vi "RT Loop - Watchdog.vi"(10 "FPGA VI Reference":T1, 11 "Message Queue":refnum<queue>) -> ()   [LabVIEW 2018]
uses:
  support/Message Queue/Message Cluster.ctl
  controls/FPGA VI Reference.ctl
  Globals/Global - Configuration Options.vi
  <vilib>/Utility/error.llb/Error Cluster From Error Code.vi
  <vilib>/rvi/errors/niLvFpgaAdjustHostInterfaceError.vi
  Globals/Global - All RT Loop Stop.vi
  <vilib>/rvi/interface/nirviReadWriteControl/nirviReadWriteControl.xnode
  NiFpgaLv.dll
  <vilib>/rvi/interface/Simulation/niFpgaSimulationCallBeginRW.vi
  support/Message Queue/Message Queue.lvlib
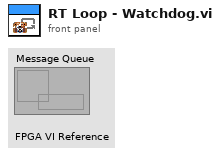
[diagram p1: front panel]
types:
  T1 = typedef "FPGA VI Reference.ctl" = refnum<k20>
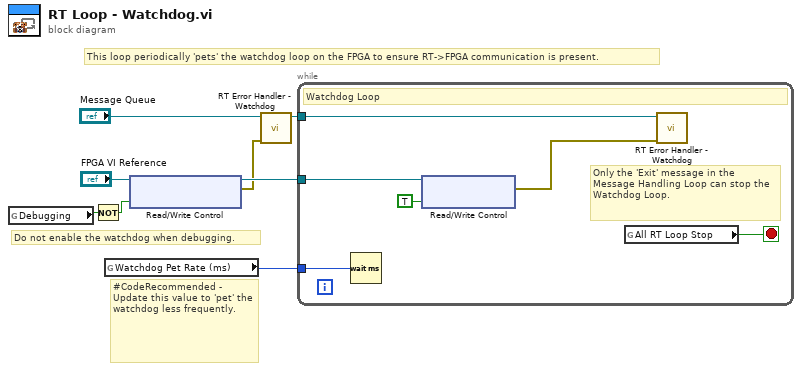
[diagram p0: block diagram]
diagram:
  # "Do not enable the watchdog when debugging."
  # "#CodeRecommended - Update this value to 'pet' the watchdog less frequently."
  # "This loop periodically 'pets' the watchdog loop on the FPGA to ensure RT->FPGA communication is present."
  n1 = global read "Global - Configuration Options.vi" "Debugging"() -> (w2:bool)
  n2 = Not(x=w2) -> (.not. x?=w1:bool)
  n3 = global read "Global - Configuration Options.vi" "Watchdog Pet Rate (ms)"() -> (w8:u32)
  n4 = xnode "Read/Write Control"("FPGA VI Reference In"="FPGA VI Reference", "Enable Watchdog"=w1) -> ("FPGA VI Reference Out"=w6:T1, "error out"=w3:errorcluster)  [unwired: 1 in]
  n5 = call "RT Error Handler - Watchdog.vi"("error in (no error)"=w3, "Message Queue"="Message Queue") -> ("dup Message Queue"=w4:refnum<queue>)  [unwired: 9 in]
  n6 = while {
    tunnel: w4 -> [w11]
    tunnel: w6 -> [w14]
    tunnel: w8 -> [w9]
    stop <- w12 stop-if-true
    # "Only the 'Exit' message in the  Message Handling Loop can stop the Watchdog Loop."
    # "Watchdog Loop"
    n7 = Wait (ms)(milliseconds to wait=w9) -> ()  [unwired: 1 out]
    n8 = xnode "Read/Write Control"("FPGA VI Reference In"=w14, "Pet Watchdog"=TRUE ("Pet RT Watchdog")) -> ("error out"=w10:errorcluster)  [unwired: 1 in, 1 out]
    n9 = global read "Global - All RT Loop Stop.vi" "All RT Loop Stop"() -> (w12:bool)
    n10 = call "RT Error Handler - Watchdog.vi"("error in (no error)"=w10, "Message Queue"=w11) -> ()  [unwired: 9 in, 1 out]
  }
